vi "Tosca-2P-Compute Sample Offset.vi"(0 "AO Fs (Hz)":dbl=100000.0, 11 "error in (no error)":errorcluster) -> (4 "x*y":i32, 8 "Offset":i32, 15 "error out":errorcluster)   [LabVIEW 2020]
uses:
  Tosca-2P-Globals.vi
panel:
  in  "DO Fs (Hz)":dbl
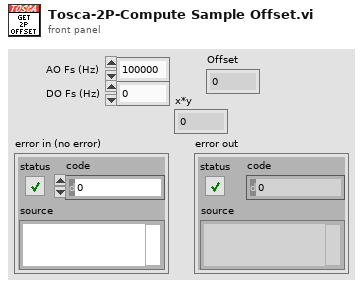
[diagram p1: front panel]
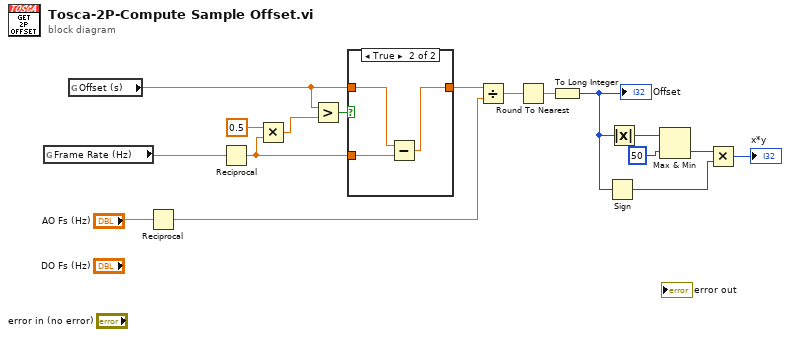
[diagram p0: block diagram]
diagram:
  n1 = global read "Tosca-2P-Globals.vi" "Frame Rate (Hz)"() -> (w17:dbl)
  n2 = global read "Tosca-2P-Globals.vi" "Offset (s)"() -> (w13:dbl)
  n3 = Reciprocal(x="AO Fs (Hz)") -> (1/x=w10:dbl)
  n4 = Reciprocal(x=w17) -> (1/x=w7:dbl)
  n5 = Multiply(x=0.5 ("y"), y=w7) -> (x*y=w14:dbl)
  n6 = Greater?(x=w13, y=w14) -> (0:w15:bool)
  n7 = case shown="True" w15 {
    tunnel: w13 -> [w18 w21]
    tunnel: [w18 w20] -> w11
    tunnel: w7 -> [_ w19]
    frame False {
    }
    frame True {
      n8 = Subtract(x=w21, y=w19) -> (x-y=w20:dbl)
    }
  }
  n9 = Divide(x=w11, y=w10) -> (x/y=w9:dbl)
  n10 = Round To Nearest(number=w9) -> (nearest integer value=w8:dbl)
  n11 = To Long Integer(number=w8) -> (32bit integer=w4:i32)
  "Offset" <- w4
  n12 = Sign(1:w4) -> (0:w2:i32)
  n13 = Absolute Value(x=w4) -> (abs(x)=w6:i32)
  n14 = Max & Min(x=w6, y=50) -> (min(x,y)=w3:i32)  [unwired: 1 out]
  n15 = Multiply(x=w3, y=w2) -> (x*y=→"x*y":i32)
